vi "Panel Data_File_Init DPT.vi"(0 "Data File Directory":path=path "c:/data", 1 "Test_Title Per TR:":string="HeatUP", 2 "Test Station:":string="1A", 3 "Scale Com Port":refnum<visa-resource-name>="COM1", 5 "Test_Type:":string="HeatUP", 7 "Version In:":string="DGnn", 9 "Supply Voltage:":string(combo), 10 "Flow Computer Info Baro,BTUF,u,Z":string[][](array[string]), 11 "error in (no error)":errorcluster, 12 "File Extension:":string="tmp", 13 "Ambient Temp SetPoint:":string="70") -> (4 "FileName":path, 6 "Header Data Array":string[][](array[string]), 8 "Nominal Load  Weight":string(combo), 14 "Weights Out":T1={"Measured IMC"=7.0, "Actual RMC"=7.0, "RMC (Desired)"=100.0, "Bone Dry Wt(lbs)"=7.0, "Tolerance(%)"=5.0} {"Tolerance(%)" format="%0#_6g"; "Bone Dry Wt(lbs)" format="%03_6g"; "RMC (Desired)" format="%0#_6g"; "Actual RMC" format="%03_6g"; "Measured IMC" format="%0#_6g"}, 15 "error out":errorcluster)   [LabVIEW 2012]
uses:
  Global Test Variables DPT.vi
  <vilib>/Utility/file.llb/Write To Spreadsheet File (string).vi
panel:
  in  "Tab Control 2":enum32{"Test Information"}(tab)
  in  "Model:":string="DGnn"
  in  "Engineer:":string="CraigT."
  in  "Technician:":string
  in  "Comments:":string
  in  "Lab ID:":string="DGnn"
  in  "TR Number:":string="T000000"
  in  "Load Run Number:":string="001"
  in  "Exhaust:":string(combo)="NR"
  in  "Drying Cycle:":string(combo)
  in  "OK":bool
  in  "Serial Number:":string="DGnn"
  in  "Ambient RH:":string="50"
  in  "Build:":string(combo)
  in  "Heat Setting:":string
  in  "Dryness Setting:":string
  in  "Frequency:":string="60 HZ"
  in  "Washer Water \nTemperature ( 60 ± 5°F ):":string="60"
  in  "Tab Control":enum32{"Location Data", "Output Data"}(tab)
  out "Unhandled Error":errorcluster
  out "Filename":string
  in  "Load Definition File":path=path "c:/Work/Loads.ini"
  out "Version:":string="DGnn"
  out "Computer:":string="1A"
  out "Load Type":string(combo)
  out "Empty Dryer Cold Weight":string="HeatUP"
  out "Date:":string="DGnn"
  out "Dryer Type:":string(combo)
  # "Filename Generated"
  # "Trrrrrrrr_uuuuuuuu_WWlb_LLLLLL_aham_xxIMC_tsid_dlr_run nnn_yyyymmdd_hhmm_DPT\nWhere:\nTrrrrrrrr - 8 digit TR #, left padded with 0's\nuuuuuuuu - is LabID number\nWW - Nom Weight\nLLLLLL - Load Type\naham - Restriction\nxx - Nom IMC\ntsid - Test Station\ndlr - Technician\nnnn - Test #\n70 - Nom Ambient Temp\n50 - Nom Ambient RH\nyyyymmddhhmm - day, month as 3 chars, 4 digit year(automatic)\nhhmm - hour and minute (24 hr) test started (automatic)\nDPT - Test Type"
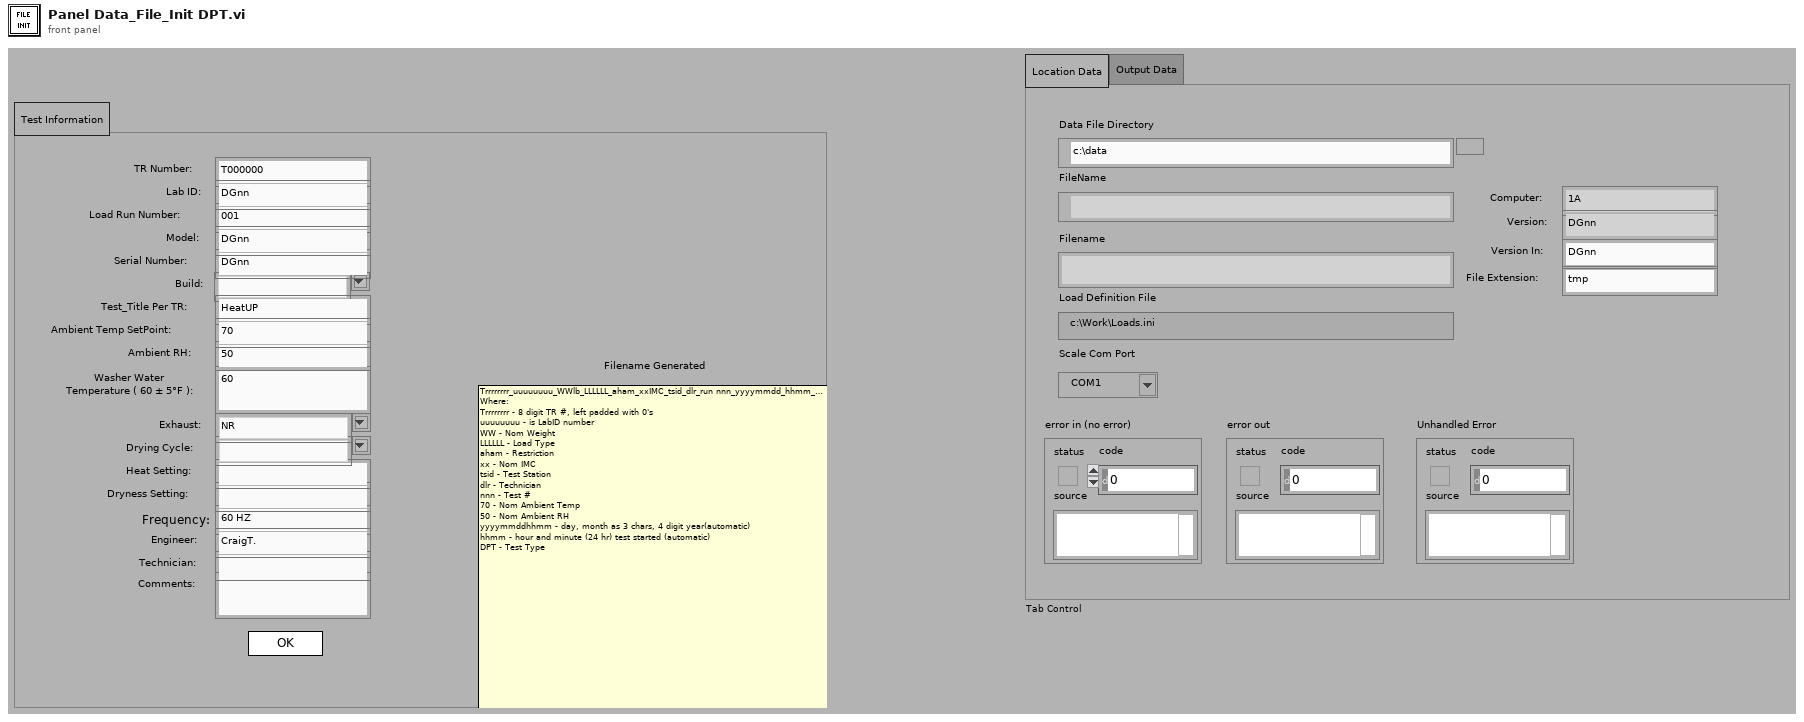
[diagram p1: front panel]
types:
  T1 = cluster{"Measured IMC":dbl, "Actual RMC":dbl, "RMC (Desired)":dbl, "Bone Dry Wt(lbs)":dbl, "Tolerance(%)":dbl}
  T2 = enum32{"invalid app kind", "Development System", "Run Time System", "Student Edition", "Embedded LabVIEW", "Evaluation", "Custom"}
  T3 = enum32{"Invalid", "Standard", "Closed", "Hidden", "Minimized", "Maximized"}
  T4 = cluster{"Core":cluster{"Current VI Reference":refnum<vi>, "Close Panel on Exit?":bool}, "Error Flag":bool, "Weights":cluster{"Measured IMC":dbl, "Actual RMC":dbl, "RMC (Desired)":dbl, "Bone Dry Wt(lbs)":dbl, "Tolerance(%)":dbl}, "Local?":bool}
  T5 = cluster{"Current VI Reference":refnum<vi>, "Close Panel on Exit?":bool}
  T6 = typedef "DPT Global Type.ctl" = cluster{"Test Setup":cluster{"RH Resistor":dbl, "Temp Cal":dbl, "Temp Coeff":dbl, "Power On Threshold":dbl, "MA Filter Size":i32, "Weight Offset":dbl, "Temp Resistor":dbl, "Gas Enabled":bool, "Gas P. Resistor":dbl, "Scale Com":dbl, "W. Samps":i32, "Temp4mA Val":dbl, "Temp20mA Val":dbl, "RH4mA Val":dbl, "RH20mA Val":dbl, "GPres4mA Val":dbl, "Gpres20mA Val":dbl, "Smoothing":bool, "CDAQ":bool, "34970":bool, "34980":bool, "RH-IP":string, "RH-IP2":string, "RH-IP3":string, "CompVolume":dbl, "T45_Coeff.":dbl}, "Agilent Setup":cluster{"Scale Channel":string, "TC Channels":string, "VDC Discrete Channels":string, "RH Chan":string, "Temp Chan":string, "Tscale Channel":string, "RDB Channel":string, "Gas Temperature":string, "Gas Pressure":string, "Barometric Pressure":string, "Gas Feedback Chan":string}, "Directories":cluster{"Work File Directory":path, "Save File Directory":path, "Library Directory":path, "Data Backup Directory":path, "Data Backup Dir Fail":path, "Lab Directory":path}, "Test Information":cluster{"Model:":string, "Temperature:":string, "Engineer:":string, "Technician:":string, "Comments:":string, "Lab ID:":string, "TR Number:":string, "Test Number:":string, "Test Station:":string, "Empty Dryer Cold Weight:":dbl, "Serial Number:":string, "Build:":string, "Dryer Type":string, "Humidity":string, "Test Title per TR:":string}, "cDAQ Array Locations":cluster{"Scale Channel":string, "TC Channels":string, "VDC Discrete Channel":string, "RH Chan":string, "Temp Chan":string, "Tscale Channel":string, "RDB Channel":string, "Gas Temperature":string, "Gas Pressure":string, "Barometric Pressure":string, "Gas Feedback Chan":string}}
  T7 = cluster{"Model:":string, "Temperature:":string, "Engineer:":string, "Technician:":string, "Comments:":string, "Lab ID:":string, "TR Number:":string, "Test Number:":string, "Test Station:":string, "Empty Dryer Cold Weight:":dbl, "Serial Number:":string, "Build:":string, "Dryer Type":string, "Humidity":string, "Test Title per TR:":string}
  T8 = typedef "DOE Audit Data.ctl" = cluster{"Technician":string, "Date":string, "Model":string, "Serial":string, "Total Dry Time(m)":dbl, "Bone Dry Wt":dbl, "Initial Wt":dbl, "Final Wt":dbl, "Initial Ret":dbl, "Final Ret":dbl, "Elect Energy Used":dbl, "Gas Meter Temp":dbl, "Gas Meter Pres":dbl, "Gas Volume":dbl, "Barometer Temp":dbl, "Barometer Pres":dbl, "Gas Corr Fact":dbl, "Cor Gas Vol":dbl, "Gas Heat Val":dbl, "Gas Energy BTU":dbl, "Gas Energy kwh 4%":dbl, "Elect Energy kwh 4%":dbl, "Total  Energy 4%":dbl, "Gas Vol Init":dbl, "Gas Vol Fin":dbl, "Start Time(s)":dbl, "End Time(s)":dbl, "Elect Energy Start":dbl, "Elect Energy End":dbl, "Per Cycle Efficency":dbl, "Annual Consumption":dbl, "Load Cycles":string, "Ambinet Temp":string, "Ambinet RH":string, "Per Cycle Off Mode/Standby Power":dbl, "Total Energy (Gas + Elect)":dbl, "Combined Energy Factor":dbl, "Off Mode Power":dbl, "Exhaust":string, "Washer Water Temperature ( 60 ± 5°F )":string, "Supply Voltage":string, "Reference Temperature (F)":string, "Reference Pressure (psi)":string, "Standby Power":dbl}
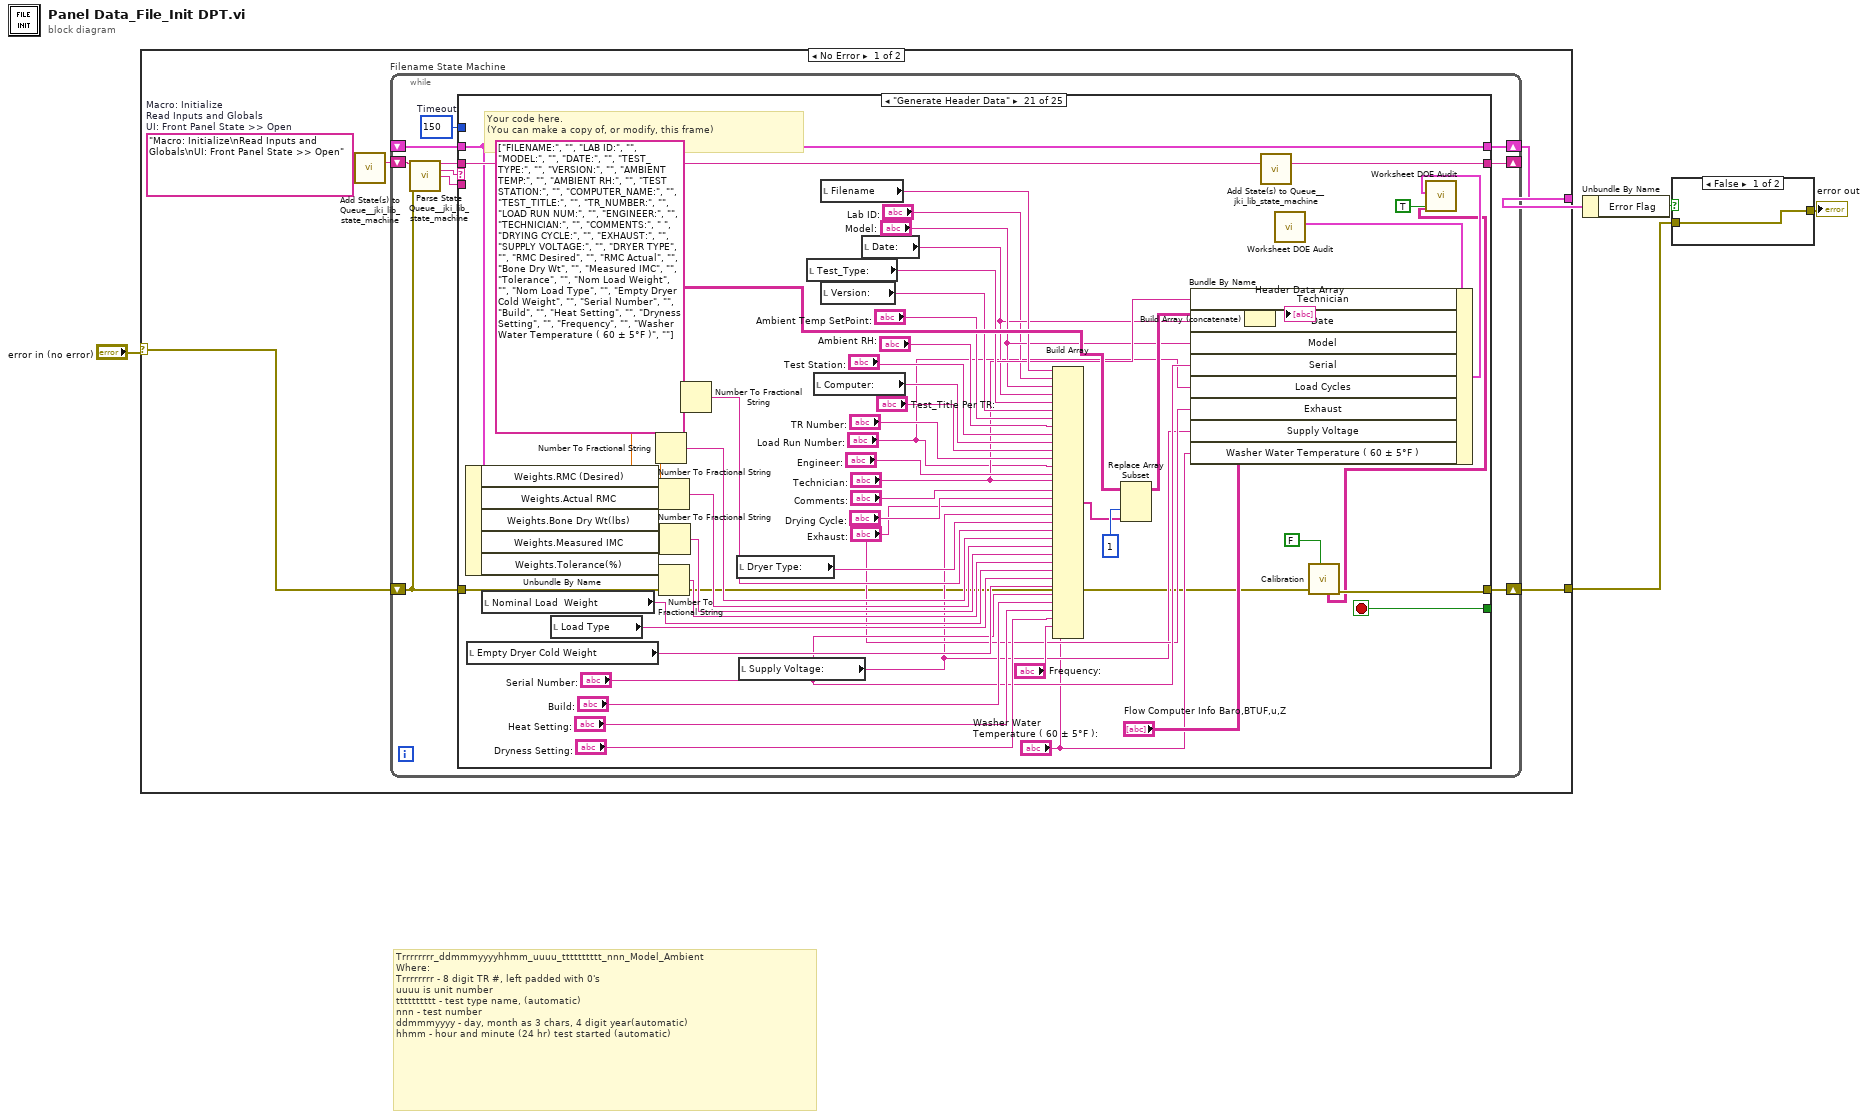
[diagram p0: block diagram]
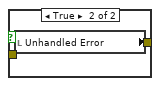
[diagram p2: hidden frame]
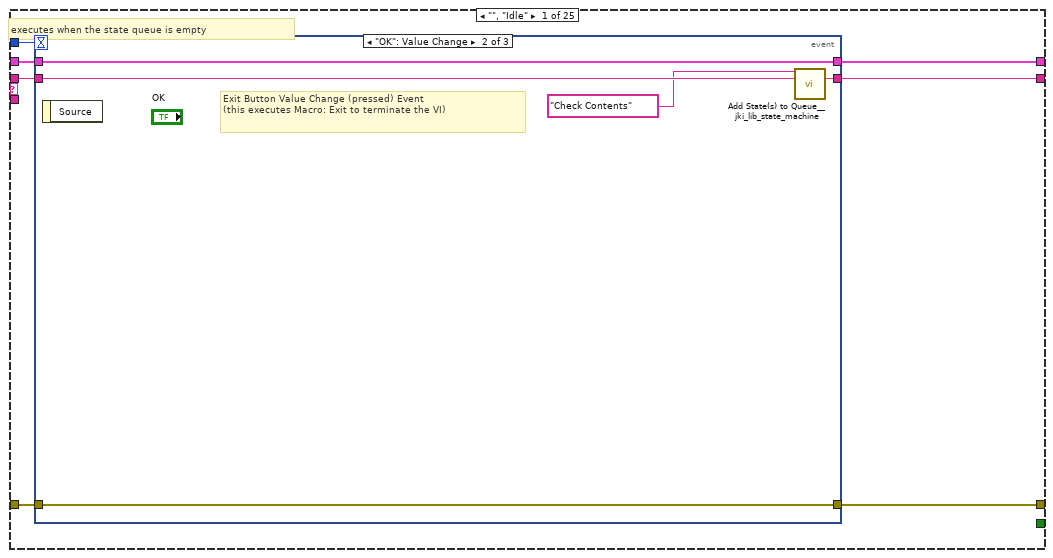
[diagram p3: hidden frame]
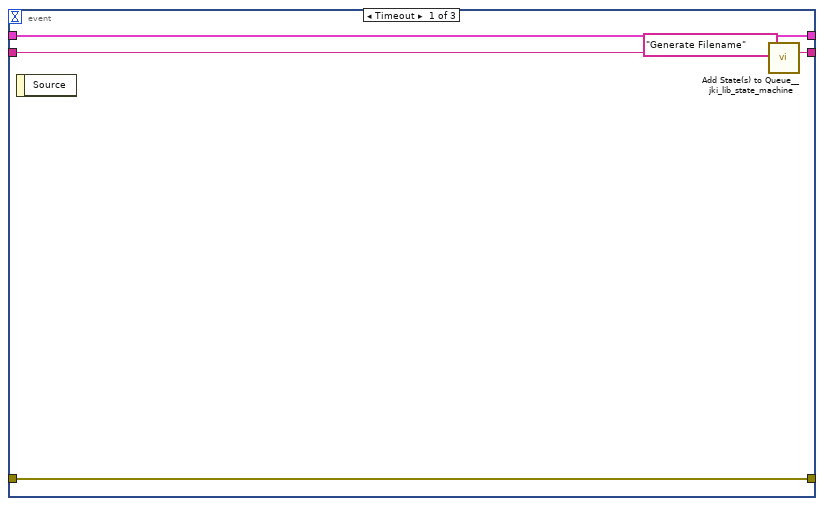
[diagram p4: hidden frame]
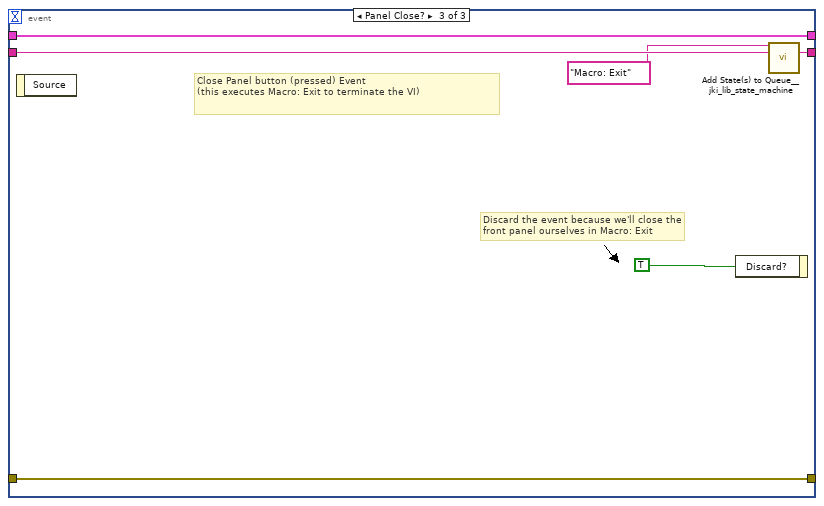
[diagram p5: hidden frame]
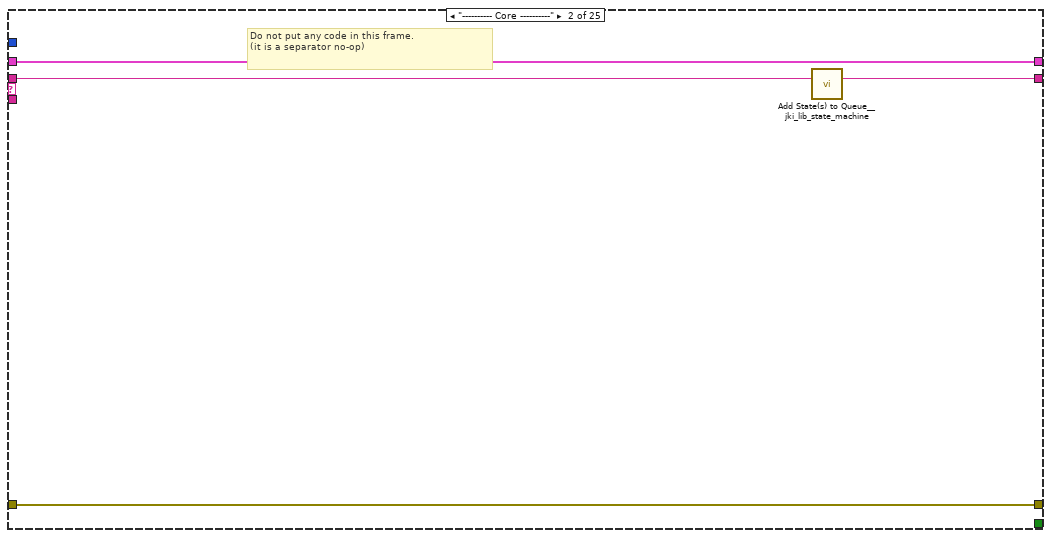
[diagram p6: hidden frame]
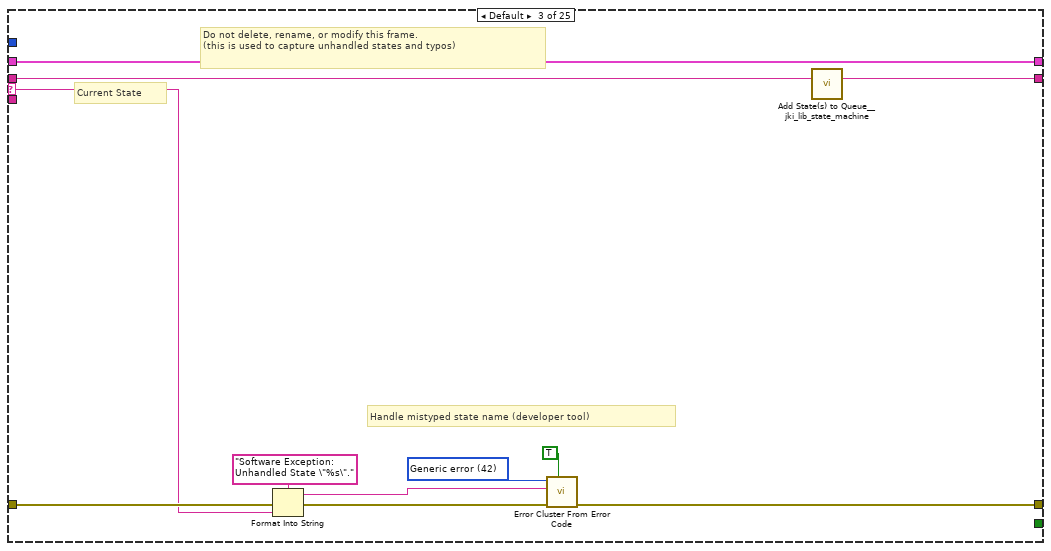
[diagram p7: hidden frame]
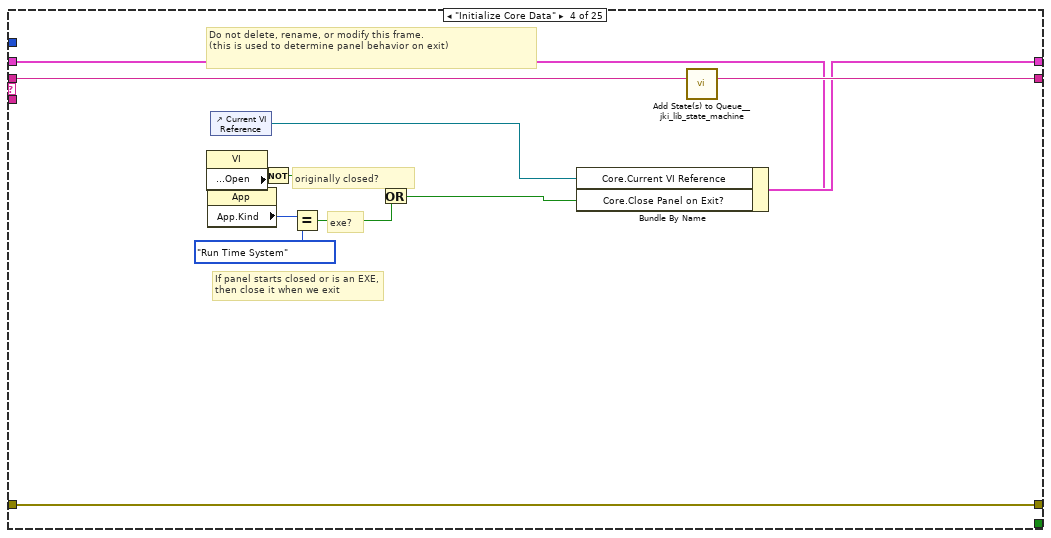
[diagram p8: hidden frame]
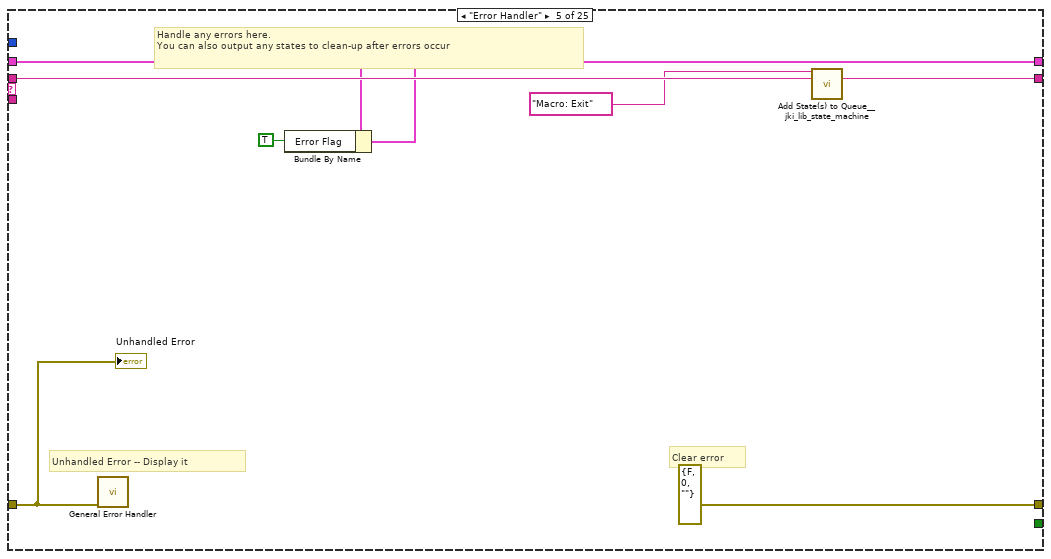
[diagram p9: hidden frame]
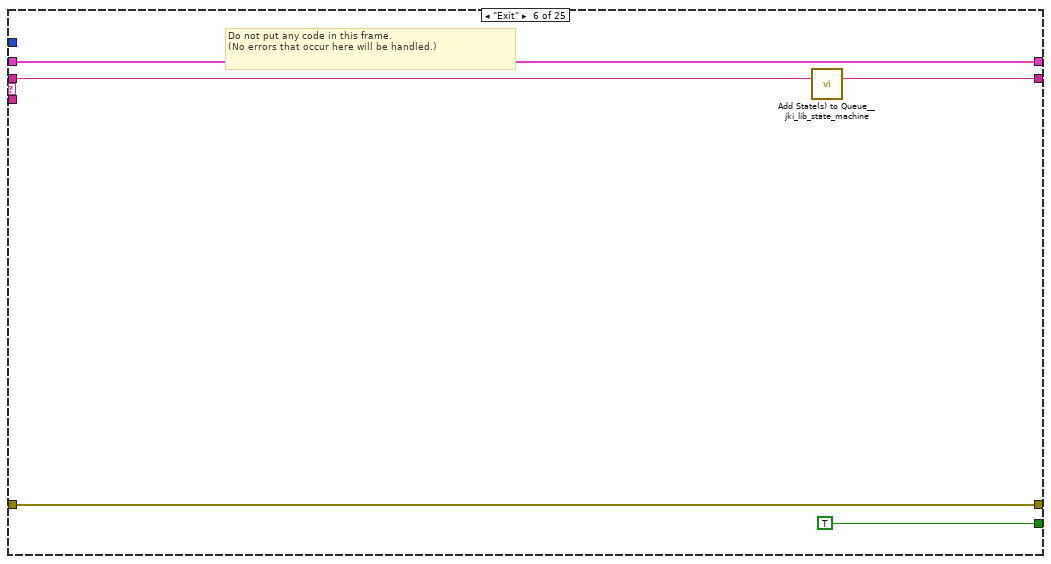
[diagram p10: hidden frame]
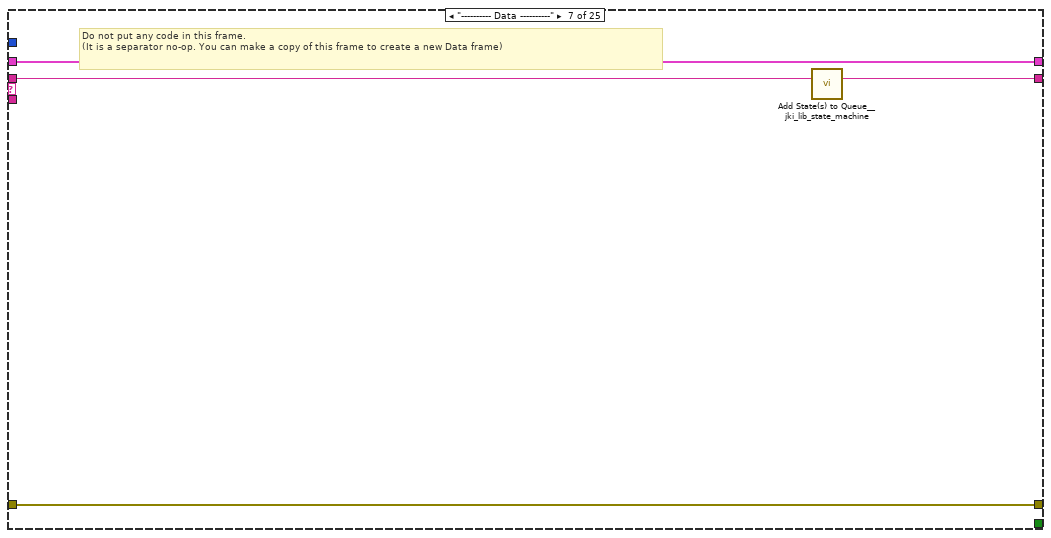
[diagram p11: hidden frame]
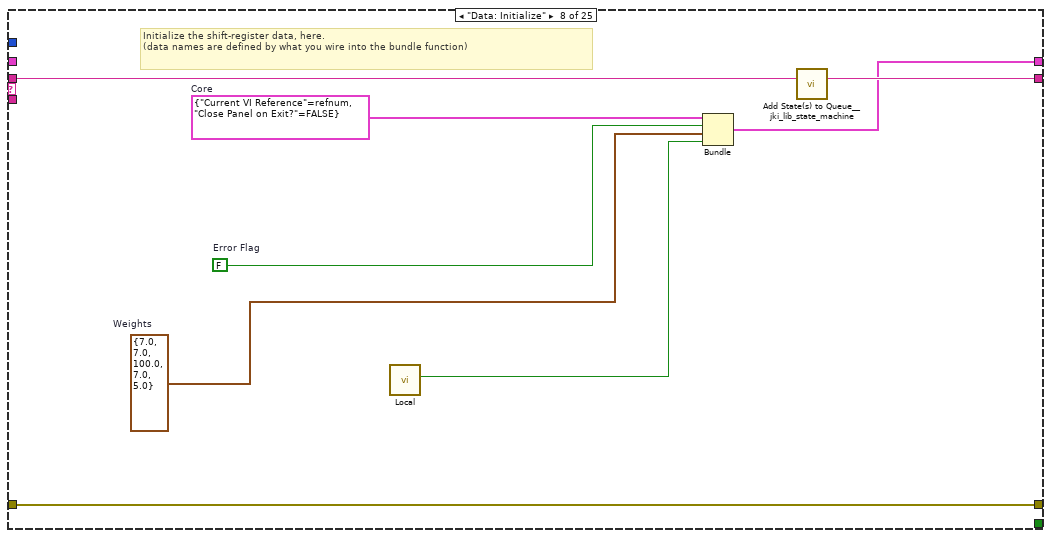
[diagram p12: hidden frame]
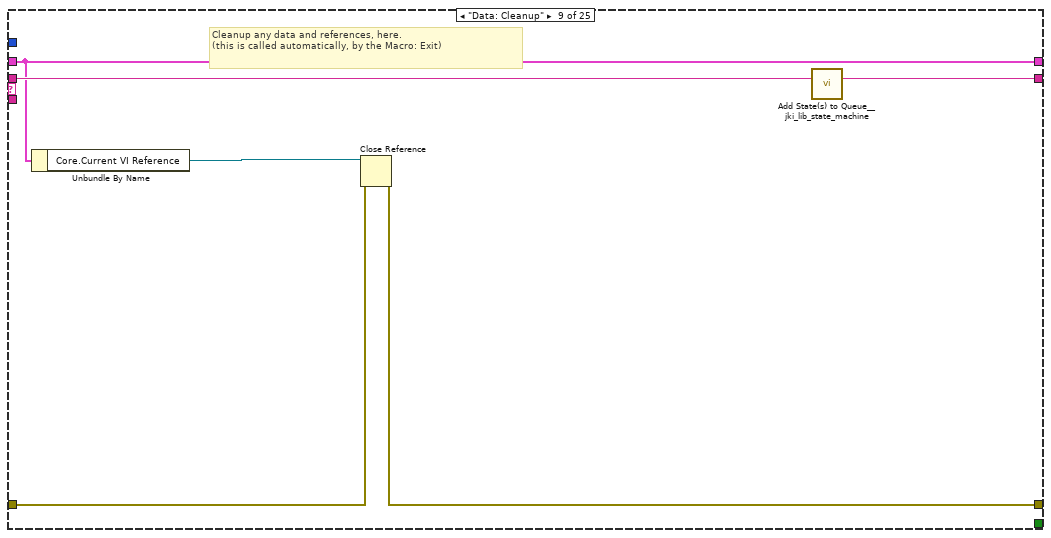
[diagram p13: hidden frame]
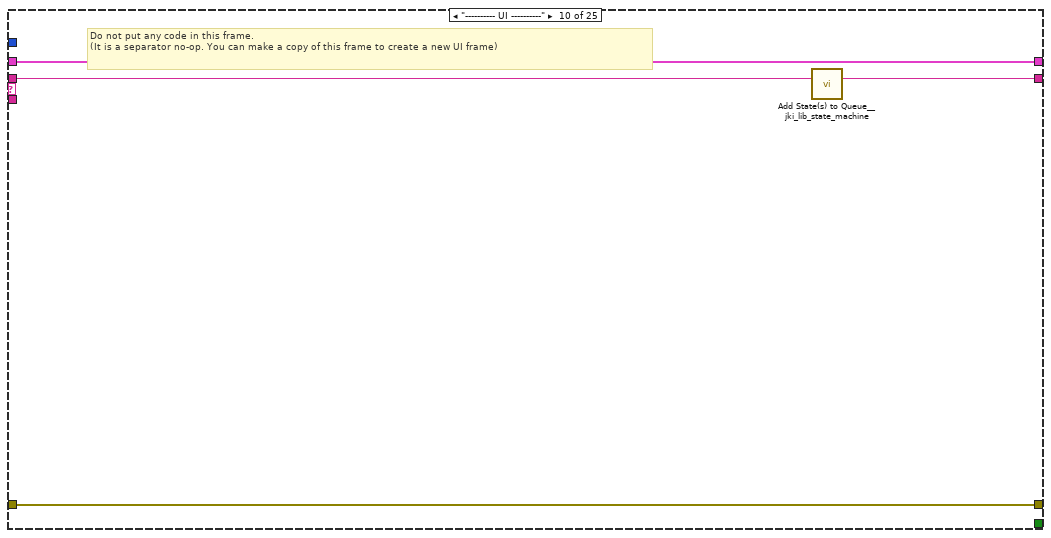
[diagram p14: hidden frame]
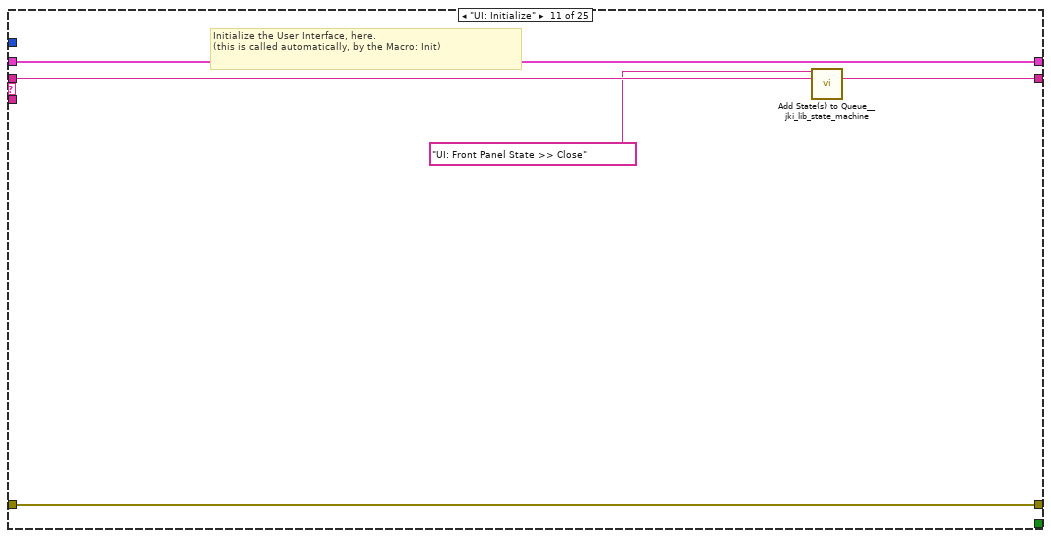
[diagram p15: hidden frame]
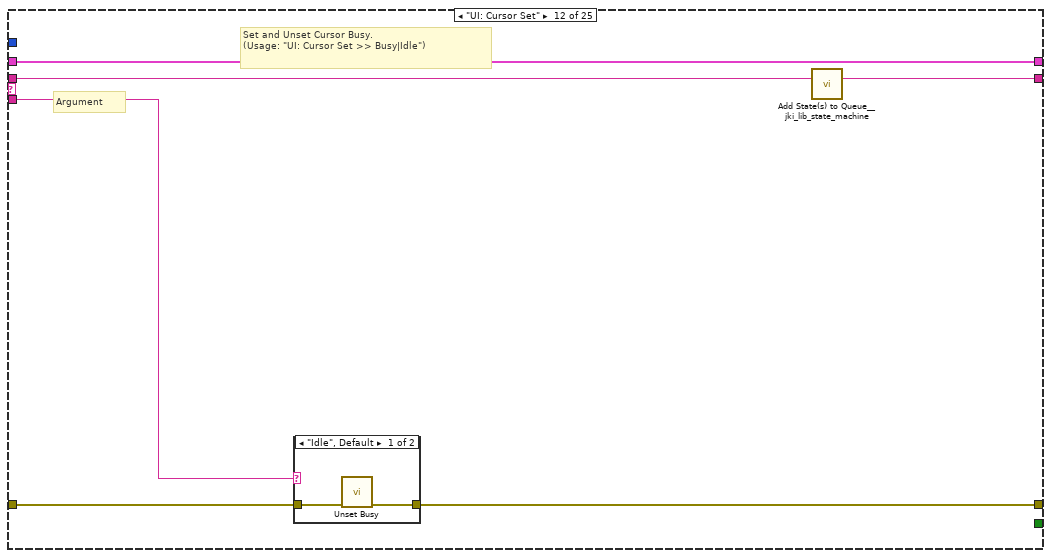
[diagram p16: hidden frame]
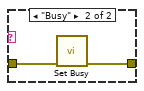
[diagram p17: hidden frame]
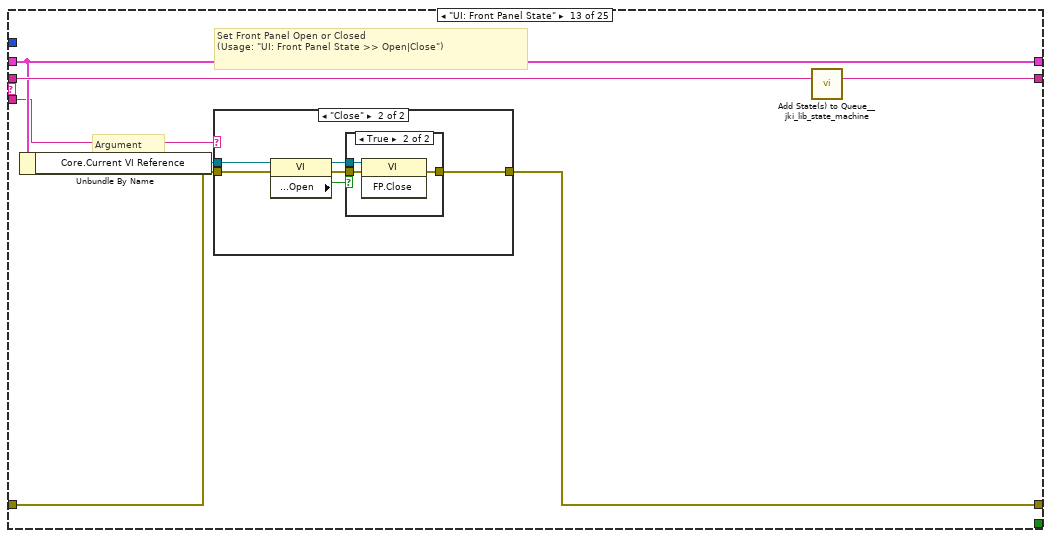
[diagram p18: hidden frame]
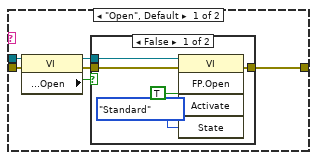
[diagram p19: hidden frame]
diagram:
  # "Trrrrrrrr_ddmmmyyyyhhmm_uuuu_tttttttttt_nnn_Model_Ambient\nWhere:\nTrrrrrrrr - 8 digit TR #, left padded with 0's\nuuuu is unit number\ntttttttttt - test type name, (automatic)\nnnn - test number\nddmmmyyyy - day, month as 3 chars, 4 digit year(automatic)\nhhmm - hour and minute (24 hr) test started (automatic)"
  n1 = case shown="No Error" "error in (no error)" {
    selector: "error in (no error)" -> [w7 w377]
    tunnel: [w8 _] -> w4
    tunnel: [w6 w377] -> w1
    frame No Error {
      w9 = "Macro: Initialize\nRead Inputs and Globals\nUI: Front Panel State >> Open"  # Macro: Initialize Read Inputs and Globals UI: Front Panel State >> Open
      n2 = call <vilib>:"Add State(s) to Queue__jki_lib_state_machine.vi"("State(s) in (\"\")"=w9) -> ("States Out"=w10:string)  [unwired: 14 in]
      n3 = while "Filename State Machine" {
        shift-right: [w14] -> w8
        shift-left: _ -> [w13]
        shift-right: [w17] -> w6
        shift-left: w7 -> [w11]
        shift-right: [w16] -> _
        shift-left: w10 -> [w18]
        stop <- w15 stop-if-true
        w12 = 150  # Timeout
        n4 = call <vilib>:"Parse State Queue__jki_lib_state_machine.vi"("State Queue"=w18, "Error In (no error)"=w11) -> ("Remaining States"=w20:string, "Current State"=w21:string, "Arguments"=w19:string)  [unwired: 11 in]
        n5 = case shown="\"Generate Header Data\"" w21 {
          selector: w21 -> [_ _ w49 _ _ _ _ _ _ _ _ _ _ _ _ _ _ _ _ _ _ _ _ _ _]
          tunnel: w20 -> [w28 w48 w53 w71 w79 w84 w88 w96 w102 w106 w111 w117 w128 w154 w163 w175 w179 w205 w225 w256 w315 w326 w353 w369 w376]
          tunnel: w19 -> [_ _ _ _ _ _ _ _ _ _ _ w112 w122 _ _ _ _ _ _ _ _ _ _ _ _]
          tunnel: w13 -> [w26 w45 w51 w62 w74 w82 w85 _ w97 w103 w109 w115 w124 w151 w160 w172 w176 w202 w222 w254 w300 w323 w340 w366 w371]
          tunnel: [w25 w46 w55 w68 errorcluster {"status"=FALSE, "code"=0, "source"=""} ("error out") w81 w86 w93 w98 w104 w108 w113 w125 w152 w161 w173 w177 w203 w223 w232 w263 w324 w351 w367 w374] -> w17
          tunnel: w11 -> [w24 w46 w54 w68 w76 w81 w86 w93 w99 w104 w108 w114 w126 w152 w161 w173 w177 w203 w223 w233 w264 w324 w351 w367 w374]
          tunnel: [w27 w47 w52 w70 w78 w83 w87 w95 w101 w105 w110 w116 w127 w153 w162 w174 w178 w204 w224 w255 w314 w325 w352 w368 w375] -> w16
          tunnel: [_ _ _ _ _ TRUE _ _ _ _ _ _ _ _ _ _ _ _ _ _ _ _ _ _ _] -> w15
          tunnel: [w23 w45 w51 w69 w73 w82 w85 w94 w97 w103 w109 w115 w124 w151 w160 w172 w176 w202 w222 w254 w300 w323 w340 w365 w371] -> w14
          tunnel: w12 -> [w22 _ _ _ _ _ _ _ _ _ _ _ _ _ _ _ _ _ _ _ _ _ _ _ _]
          frame "", "Idle" {
            # "executes when the state queue is empty"
            n6 = event shown="[1] \"OK\": Value Change" {
              selector: _ -> [_ _ _]
              dyn-events: _ -> [_ _ _]
              timeout: w22 -> [_ _ _]
              tunnel: w28 -> [w33 w38 w44]
              tunnel: [w32 w37 w43] -> w27
              tunnel: w26 -> [w30 w35 w41]
              tunnel: [w31 w36 w42] -> w25
              tunnel: w24 -> [w31 w36 w42]
              tunnel: [w30 w35 w41] -> w23
              event Timeout {
                n7 = event-data() -> ()  [unwired: 1 in, 1 out]
                n8 = call <vilib>:"Add State(s) to Queue__jki_lib_state_machine.vi"("State(s) in Front (\"\")"="Generate Filename" ("State(s) in Front (\"\")"), "State(s) in (\"\")"=w33) -> ("States Out"=w32:string)  [unwired: 13 in]
              }
              event "OK": Value Change {
                # "Exit Button Value Change (pressed) Event\n(this executes Macro: Exit to terminate the VI)"
                n9 = event-data() -> ()  [unwired: 1 in, 1 out]
                n10 = call <vilib>:"Add State(s) to Queue__jki_lib_state_machine.vi"("State(s) in Front (\"\")"="Check Contents", "State(s) in (\"\")"=w38) -> ("States Out"=w37:string)  [unwired: 13 in]
              }
              event Panel Close? {
                # "Discard the event because we'll close the front panel ourselves in Macro: Exit"
                # "Close Panel button (pressed) Event\n(this executes Macro: Exit to terminate the VI)"
                n11 = event-data() -> ()  [unwired: 1 in, 1 out]
                n12 = event-data("Discard?"=TRUE) -> ()  [unwired: 1 in, 1 out]
                n13 = call <vilib>:"Add State(s) to Queue__jki_lib_state_machine.vi"("State(s) in Front (\"\")"="Macro: Exit", "State(s) in (\"\")"=w44) -> ("States Out"=w43:string)  [unwired: 13 in]
              }
            }
          }
          frame "---------- Core ----------" {
            # "Do not put any code in this frame.\n(it is a separator no-op)"
            n14 = call <vilib>:"Add State(s) to Queue__jki_lib_state_machine.vi"("State(s) in (\"\")"=w48) -> ("States Out"=w47:string)  [unwired: 14 in]
          }
          frame Default {
            w58 = 42 items=["No error", "Argument error", "Memory is full", "Out of zone", "End of file", "File already open", "Generic file I/O error", "File not found", "File permission error", "Disk is full", "Duplicate path", "Too many files open", "System feature not enabled", "Resource file not found", "Cannot add resource", "Resource not found", "Image not found", "Image memory error", "Pen does not exist", "Config type invalid", "Config token not found", "Config parse error", "Config memory error", "Bad external code format", "Bad external code offset", "External code not present", "Null window", "Destroy window error", "Null menu", "Print aborted", "Bad print record", "Print driver error", "Windows error during printing", "Memory error during printing", "Print dialog error", "Generic print error", "Invalid device refnum", "Device not found", "Device parameter error", "Device unit error", "Cannot open device", "Device call aborted", "Generic error", "Cancelled by user", "Object ID too low", "Object ID too high", "Object not in heap", "Unknown heap", "Unknown object (invalid DefProc)", "Unknown object (DefProc not in table)", "Message out of range", "Invalid (null) method", "Unknown message", "Manager call not supported", "Bad address", "Network operation in progress", "Network operation timed out", "Connection is busy", "Network attribute not supported", "Network error", "Address in use", "System out of memory", "Connection aborted", "Connection refused", "Not connected", "Already connected", "Connection closed", "Initialization error (interapplication manager)", "Bad occurrence", "Wait on unbound occurrence handler", "Occurrence queue overflow", "Datalog type conflict", "Unused", "Unrecognized type (interapplication manager)", "Memory corrupt", "Failed to make temporary DLL", "Old CIN version", "Drag socket not found", "Failed to load drop-object", "Failed to register OLE object", "Failed to release OLE object", "Format specifier type mismatch", "Unknown format specifier", "Too few format specifiers", "Too many format specifiers", "Scan failed", "Newer CIN version", "Error converting to variant", "Runtime menu error", "Password tampered", "Variant attribute not found", "Incompatible variant data type", "Event data is not available", "Event Store is not present", "Occurrence is not found", "Event Queue is not created", "Event info is not available", "Refnum passed is NULL", "Error retrieving Class GUID", "Error retrieving CoClass GUID", "Error retrieving TypeLib GUID.", "Bad built application magic bytes.", "Specific driver is different from the specific driver associated with the Logical Name.", "There is no session opened to the class driver.", "Max Error", "MAX - Error with config objects", "MAX - Error loading configuration", "MAX - Group not supported"]
            # "Current State"
            # "Do not delete, rename, or modify this frame.\n(this is used to capture unhandled states and typos)"
            # "Handle mistyped state name (developer tool)"
            n15 = Format Into String(format string="Software Exception: Unhandled State \"%s\"." ("message"), error in=w54, w49) -> (resulting string=w57:string, error out=w56:errorcluster)  [unwired: 1 in]
            n16 = call <vilib>:"Error Cluster From Error Code.vi"("show call chain? (False)"=TRUE, "error in (no error)"=w56, "error message (\"\")"=w57, "error code (0)"=w58) -> ("error out"=w55:errorcluster)  [unwired: 5 in]
            n17 = call <vilib>:"Add State(s) to Queue__jki_lib_state_machine.vi"("State(s) in (\"\")"=w53) -> ("States Out"=w52:string)  [unwired: 14 in]
          }
          frame "Initialize Core Data" {
            # "Do not delete, rename, or modify this frame.\n(this is used to determine panel behavior on exit)"
            # "originally closed?"
            # "exe?"
            # "If panel starts closed or is an EXE, then close it when we exit"
            n18 = property class="VI"() -> ("Front Panel.Open"=w67:bool)  [unwired: 2 in, 2 out]
            n19 = property class="App"() -> ("App.Kind"=w66:T2)  [unwired: 2 in, 2 out]
            n20 = control-ref of="Current VI Reference"() -> (w60:refnum<vi>)
            n21 = Not(x=w67) -> (.not. x?=w64:bool)
            n22 = Equal?(x=w66, y=T2."Run Time System" ("Application:Kind")) -> (x = y?=w63:bool)
            n23 = Or(x=w64, y=w63) -> (x .or. y?=w61:bool)
            n24 = Bundle By Name(cluster=w62, "Core.Current VI Reference"=w60, "Core.Close Panel on Exit?"=w61) -> (w69:T4)
            n25 = call <vilib>:"Add State(s) to Queue__jki_lib_state_machine.vi"("State(s) in (\"\")"=w71) -> ("States Out"=w70:string)  [unwired: 14 in]
          }
          frame "Error Handler" {
            # "Unhandled Error -- Display it"
            # "Handle any errors here.\nYou can also output any states to clean-up after errors occur"
            # "Clear error"
            n26 = call <vilib>:"General Error Handler.vi"("error in (no error)"=w76) -> ()  [unwired: 10 in, 5 out]
            n27 = Bundle By Name(cluster=w74, "Error Flag"=TRUE) -> (w73:T4)
            n28 = call <vilib>:"Add State(s) to Queue__jki_lib_state_machine.vi"("State(s) in Front (\"\")"="Macro: Exit", "State(s) in (\"\")"=w79) -> ("States Out"=w78:string)  [unwired: 13 in]
            "Unhandled Error" <- w76
          }
          frame "Exit" {
            # "Do not put any code in this frame.\n(No errors that occur here will be handled.)"
            n29 = call <vilib>:"Add State(s) to Queue__jki_lib_state_machine.vi"("State(s) in (\"\")"=w84) -> ("States Out"=w83:string)  [unwired: 14 in]
          }
          frame "---------- Data ----------" {
            # "Do not put any code in this frame.\n(It is a separator no-op. You can make a copy of this frame to create a new Data frame)"
            n30 = call <vilib>:"Add State(s) to Queue__jki_lib_state_machine.vi"("State(s) in (\"\")"=w88) -> ("States Out"=w87:string)  [unwired: 14 in]
          }
          frame "Data: Initialize" {
            w90 = T1 {"Measured IMC"=7.0, "Actual RMC"=7.0, "RMC (Desired)"=100.0, "Bone Dry Wt(lbs)"=7.0, "Tolerance(%)"=5.0}  # Weights
            w91 = T5 {"Current VI Reference"=refnum, "Close Panel on Exit?"=FALSE}  # Core
            w92 = FALSE  # Error Flag
            # "Initialize the shift-register data, here.\n(data names are defined by what you wire into the bundle function)"
            n31 = call "Local.vi"() -> ("Local?"=w89:bool)  [unwired: 11 in]
            n32 = Bundle("Core"=w91, "Error Flag"=w92, "Weights"=w90, "Local?"=w89) -> (w94:T4)  [unwired: 1 in]
            n33 = call <vilib>:"Add State(s) to Queue__jki_lib_state_machine.vi"("State(s) in (\"\")"=w96) -> ("States Out"=w95:string)  [unwired: 14 in]
          }
          frame "Data: Cleanup" {
            # "Cleanup any data and references, here.\n(this is called automatically, by the Macro: Exit)"
            n34 = Unbundle By Name(w97) -> ("Core.Current VI Reference"=w100:refnum<vi>)
            n35 = Close Reference(reference=w100, error in (no error)=w99) -> (error out=w98:errorcluster)
            n36 = call <vilib>:"Add State(s) to Queue__jki_lib_state_machine.vi"("State(s) in (\"\")"=w102) -> ("States Out"=w101:string)  [unwired: 14 in]
          }
          frame "---------- UI ----------" {
            # "Do not put any code in this frame.\n(It is a separator no-op. You can make a copy of this frame to create a new UI frame)"
            n37 = call <vilib>:"Add State(s) to Queue__jki_lib_state_machine.vi"("State(s) in (\"\")"=w106) -> ("States Out"=w105:string)  [unwired: 14 in]
          }
          frame "UI: Initialize" {
            # "Initialize the User Interface, here.\n(this is called automatically, by the Macro: Init)"
            n38 = call <vilib>:"Add State(s) to Queue__jki_lib_state_machine.vi"("State(s) in Front (\"\")"="UI: Front Panel State >> Close", "State(s) in (\"\")"=w111) -> ("States Out"=w110:string)  [unwired: 13 in]
          }
          frame "UI: Cursor Set" {
            # "Argument"
            # "Set and Unset Cursor Busy.\n(Usage: \"UI: Cursor Set >> Busy|Idle\")"
            n39 = case shown="\"Idle\", Default" w112 {
              tunnel: w114 -> [w119 w121]
              tunnel: [w118 w120] -> w113
              frame "Idle", Default {
                n40 = call <vilib>:"Unset Busy.vi"("error in (no error)"=w119) -> ("error out"=w118:errorcluster)  [unwired: 10 in]
              }
              frame "Busy" {
                n41 = call <vilib>:"Set Busy.vi"("error in (no error)"=w121) -> ("error out"=w120:errorcluster)  [unwired: 9 in, 1 out]
              }
            }
            n42 = call <vilib>:"Add State(s) to Queue__jki_lib_state_machine.vi"("State(s) in (\"\")"=w117) -> ("States Out"=w116:string)  [unwired: 14 in]
          }
          frame "UI: Front Panel State" {
            # "Argument"
            # "Set Front Panel Open or Closed\n(Usage: \"UI: Front Panel State >> Open|Close\")"
            n43 = Unbundle By Name(w124) -> ("Core.Current VI Reference"=w123:refnum<vi>)
            n44 = case shown="\"Close\"" w122 {
              tunnel: w126 -> [w132 w145]
              tunnel: [w134 w146] -> w125
              tunnel: w123 -> [w133 w143]
              frame "Open", Default {
                n45 = property class="VI"(reference=w133, error in=w132) -> (reference out=w130:refnum<vi>, error out=w131:errorcluster, "Front Panel.Open"=w129:bool)
                n46 = case shown="False" w129 {
                  tunnel: [w137 w140] -> w134
                  tunnel: w131 -> [w136 w140]
                  tunnel: w130 -> [w135 _]
                  frame False {
                    n47 = invoke class="VI" method="FP.Open"(reference=w135, error in=w136, "Activate"=TRUE, "State"=T3."Standard") -> (error out=w137:errorcluster)  [unwired: 1 in, 4 out]
                  }
                  frame True {
                  }
                }
              }
              frame "Close" {
                n48 = property class="VI"(reference=w143, error in=w145) -> (reference out=w142:refnum<vi>, error out=w144:errorcluster, "Front Panel.Open"=w141:bool)
                n49 = case shown="True" w141 {
                  tunnel: [w147 w150] -> w146
                  tunnel: w144 -> [w147 w149]
                  tunnel: w142 -> [_ w148]
                  frame False {
                  }
                  frame True {
                    n50 = invoke class="VI" method="FP.Close"(reference=w148, error in=w149) -> (error out=w150:errorcluster)  [unwired: 1 in, 2 out]
                  }
                }
              }
            }
            n51 = call <vilib>:"Add State(s) to Queue__jki_lib_state_machine.vi"("State(s) in (\"\")"=w128) -> ("States Out"=w127:string)  [unwired: 14 in]
          }
          frame "---------- Macro ----------" {
            # "Do not put any code in this frame.\n(It is a separator no-op. You can make a copy of this frame to create a new Macro frame)"
            n52 = call <vilib>:"Add State(s) to Queue__jki_lib_state_machine.vi"("State(s) in (\"\")"=w154) -> ("States Out"=w153:string)  [unwired: 14 in]
          }
          frame "Macro: Initialize" {
            # "Initialization Macro\n(This is called once, when the VI starts)"
            n53 = property on="OK" class="Bool"("Key Focus"=FALSE) -> ()  [unwired: 2 in, 2 out]
            n54 = local write "Drying Cycle:"("" ("Drying Cycle:")) -> ()
            n55 = local write "Exhaust:"("" ("Exhaust:")) -> ()
            n56 = local write "Dryer Type:"("" ("Dryer Type:")) -> ()
            n57 = call <vilib>:"Add State(s) to Queue__jki_lib_state_machine.vi"("State(s) in Front (\"\")"="Data: Initialize\nInitialize Core Data\nUI: Initialize", "State(s) in (\"\")"=w163) -> ("States Out"=w162:string)  [unwired: 13 in]
          }
          frame "Macro: Exit" {
            # "Exit Macro\n(This is called once, when the VI exits)"
            n58 = Unbundle By Name(w172) -> ("Core.Close Panel on Exit?"=w171:bool, "Local?"=w164:bool)
            n59 = Compound Arithmetic op=AND(w171, invert w164) -> (w165:bool)
            n60 = Select(t="UI: Front Panel State >> Close", s=w165, f="") -> (s? t:f=w168:string)
            n61 = call <vilib>:"Add State(s) to Queue__jki_lib_state_machine.vi"("State(s) in (\"\")"=w168, "State(s) at Back (\"\")"="Data: Cleanup\nExit") -> ("States Out"=w166:string)  [unwired: 13 in]
            n62 = call <vilib>:"Add State(s) to Queue__jki_lib_state_machine.vi"("State(s) in Front (\"\")"=w166, "State(s) in (\"\")"=w175) -> ("States Out"=w174:string)  [unwired: 13 in]
          }
          frame "---------- New Category ----------" {
            # "Template Separator\n(You can make a copy of, or modify, this frame)"
            n63 = call <vilib>:"Add State(s) to Queue__jki_lib_state_machine.vi"("State(s) in (\"\")"=w179) -> ("States Out"=w178:string)  [unwired: 14 in]
          }
          frame "Read Inputs and Globals" {
            n64 = global read "Global Test Variables DPT.vi" "Globals for Dryer Performance Test"() -> (w197:T6)
            n65 = call "IP and Computer Name.vi"() -> ("Computer Name"=→"Computer:":string)  [unwired: 10 in, 1 out]
            n66 = Unbundle By Name(w197) -> ("Test Information"=w196:T7)
            n67 = Unbundle(w196) -> ("Model:"=w195:string, "Temperature:"=w187:string, "Engineer:"=w194:string, "Technician:"=w193:string, "Comments:"=w192:string, "Lab ID:"=w191:string, "TR Number:"=w190:string, "Test Number:"=w189:string, "Test Station:"=w188:string, "Empty Dryer Cold Weight:"=w184:dbl, "Serial Number:"=w186:string, "Build:"=w185:string, "Dryer Type"=→"Dryer Type:":string, "Humidity"=w181:string, "Test Title per TR:"=w180:string)
            n68 = local write "Comments:"(w192) -> ()
            n69 = local write "Technician:"(w193) -> ()
            n70 = local write "Test Station:"(w188) -> ()
            n71 = local write "Load Run Number:"(w189) -> ()
            n72 = local write "Ambient Temp SetPoint:"(w187) -> ()
            n73 = local write "Serial Number:"(w186) -> ()
            n74 = Format Date/Time String(time format string (%c)="%Y%m%d_%H%M") -> (date/time string=→"Date:":string)  [unwired: 2 out]
            n75 = local write "Test_Title Per TR:"(w180) -> ()
            n76 = local write "Lab ID:"(w191) -> ()
            n77 = local write "TR Number:"(w190) -> ()
            n78 = local write "Build:"(w185) -> ()
            n79 = local write "Ambient RH:"(w181) -> ()
            n80 = local write "Engineer:"(w194) -> ()
            n81 = local write "Model:"(w195) -> ()
            n82 = Number To Fractional String(number=w184) -> (F-format string=→"Empty Dryer Cold Weight":string)  [unwired: 3 in]
            n83 = call <vilib>:"Add State(s) to Queue__jki_lib_state_machine.vi"("State(s) in (\"\")"=w205) -> ("States Out"=w204:string)  [unwired: 14 in]
            "Version:" <- "Version In:"
          }
          frame "Write Globals" {
            # "Your code here.\n(You can make a copy of, or modify, this frame)"
            n84 = local read "Comments:"() -> (w214:string)
            n85 = local read "Technician:"() -> (w215:string)
            n86 = global read "Global Test Variables DPT.vi" "Globals for Dryer Performance Test"() -> (w211:T6)
            n87 = local read "Test_Title Per TR:"() -> (w208:string)
            n88 = local read "Serial Number:"() -> (w206:string)
            n89 = local read "TR Number:"() -> (w213:string)
            n90 = local read "Test Station:"() -> (w212:string)
            n91 = local read "Ambient RH:"() -> (w207:string)
            n92 = local read "Engineer:"() -> (w216:string)
            n93 = local read "Ambient Temp SetPoint:"() -> (w217:string)
            n94 = local read "Load Run Number:"() -> (w219:string)
            n95 = local read "Model:"() -> (w218:string)
            n96 = local read "Lab ID:"() -> (w220:string)
            n97 = Unbundle By Name(w211) -> ("Test Information"=w221:T7)
            n98 = Bundle By Name(cluster=w221, "Model:"=w218, "Temperature:"=w217, "Engineer:"=w216, "Technician:"=w215, "Comments:"=w214, "Lab ID:"=w220, "TR Number:"=w213, "Test Number:"=w219, "Test Station:"=w212, "Humidity"=w207, "Test Title per TR:"=w208, "Serial Number:"=w206) -> (w210:T7)
            n99 = Bundle By Name(cluster=w211, "Test Information"=w210) -> (w209:T6)
            n100 = global write "Global Test Variables DPT.vi" "Globals for Dryer Performance Test"(w209) -> ()
            n101 = call <vilib>:"Add State(s) to Queue__jki_lib_state_machine.vi"("State(s) in (\"\")"=w225) -> ("States Out"=w224:string)  [unwired: 14 in]
          }
          frame "Generate Filename" {
            # "Trrrrrrrr_uuuuuuuu_WWlb_LLLLLL_aham_xxIMC_tsid_dlr_run nnn_70,50_yyyymmdd_hhmm_DPT\nWhere:\nTrrrrrrrr - 8 digit TR #, left padded with 0's\nuuuuuuuu - is unit number\nWW - Nom Weight\nLLLLLL - Load Type\naham - Restriction\nxx - Nom IMC\ntsid - Test Station\ndlr - Technician\nnnn - Test #\n70 - Nom Ambient Temp\n50 - Nom Ambient RH\nyyyymmddhhmm - day, month as 3 chars, 4 digit year(automatic)\nhhmm - hour and minute (24 hr) test started (automatic)\nDPT - Test Type"
            # "Your code here.\n(You can make a copy of, or modify, this frame)"
            n102 = local read "Ambient Temp SetPoint:"() -> (w249:string)
            n103 = local read "Nominal Load  Weight"() -> (w238:string)
            n104 = local read "Load Run Number:"() -> (w248:string)
            n105 = local read "Weights Out"() -> (w245:T1)
            n106 = local read "Technician:"() -> (w247:string)
            n107 = local read "Test Station:"() -> (w246:string)
            n108 = local read "Load Type"() -> (w239:string)
            n109 = local read "TR Number:"() -> (w252:string)
            n110 = local read "Lab ID:"() -> (w237:string)
            n111 = local read "Date:"() -> (w250:string)
            n112 = local read "Exhaust:"() -> (w240:string)
            n113 = Unbundle By Name(w245) -> ("RMC (Desired)"=w244:dbl)
            n114 = Number To Fractional String(number=w244, width (-)=i16 2, precision (6)=i16 0) -> (F-format string=w243:string)  [unwired: 1 in]
            n115 = Format Into String(format string="%09s_%08s_%2.2slb_%06.6s_%04.4s_%03.3sIMC_%4.4s_%03.3s_run %3.3s_%s_%13.13s_DPT.%3.3s", w252, w237, w238, w239, w240, w243, w246, w247, w248, w249, w250, "File Extension:") -> (resulting string=w229:string)  [unwired: 2 in, 1 out]
            "Filename" <- w229
            n116 = Path To String(path="Data File Directory") -> (string=w227:string)
            n117 = Build Path(base path="Data File Directory", name or relative path=w229) -> (appended path=w235:path)
            "FileName" <- w235
            n118 = Equal?(x=w235, y=path "") -> (x = y?=w234:bool)
            n119 = Concatenate Strings("Error for Filename: " ("source"), w229, " Directory: " ("source"), w227) -> (w226:string)
            n120 = case shown="True" w234 {
              tunnel: w233 -> [w257 _]
              tunnel: [w257 w259] -> w232
              tunnel: w226 -> [_ w258]
              frame False {
              }
              frame True {
                n121 = Bundle By Name(cluster=errorcluster {"status"=TRUE, "code"=-8074, "source"=""} ("error IO"), "source"=w258) -> (w259:errorcluster)
              }
            }
            n122 = call <vilib>:"Add State(s) to Queue__jki_lib_state_machine.vi"("State(s) in (\"\")"=w256) -> ("States Out"=w255:string)  [unwired: 14 in]
          }
          frame "Generate Header Data" {
            # "Your code here.\n(You can make a copy of, or modify, this frame)"
            n123 = Unbundle By Name(w300) -> ("Weights.RMC (Desired)"=w299:dbl, "Weights.Actual RMC"=w298:dbl, "Weights.Bone Dry Wt(lbs)"=w297:dbl, "Weights.Measured IMC"=w296:dbl, "Weights.Tolerance(%)"=w291:dbl)
            n124 = local read "Empty Dryer Cold Weight"() -> (w287:string)
            n125 = local read "Nominal Load  Weight"() -> (w289:string)
            n126 = local read "Load Type"() -> (w288:string)
            n127 = Number To Fractional String(number=w298) -> (F-format string=w294:string)  [unwired: 3 in]
            n128 = Number To Fractional String(number=w297) -> (F-format string=w293:string)  [unwired: 3 in]
            n129 = Number To Fractional String(number=w291) -> (F-format string=w290:string)  [unwired: 3 in]
            n130 = Number To Fractional String(number=w296) -> (F-format string=w292:string)  [unwired: 3 in]
            n131 = Number To Fractional String(number=w299) -> (F-format string=w295:string)  [unwired: 3 in]
            n132 = local read "Dryer Type:"() -> (w283:string)
            n133 = local read "Supply Voltage:"() -> (w266:string)
            n134 = local read "Test_Type:"() -> (w309:string)
            n135 = local read "Computer:"() -> (w306:string)
            n136 = local read "Filename"() -> (w310:string)
            n137 = local read "Version:"() -> (w308:string)
            n138 = local read "Date:"() -> (w274:string)
            n139 = Build Array(w310, "Lab ID:", "Model:", w274, w309, w308, "Ambient Temp SetPoint:", "Ambient RH:", "Test Station:", w306, "Test_Title Per TR:", "TR Number:", "Load Run Number:", "Engineer:", "Technician:", "Comments:", "Drying Cycle:", "Exhaust:", w266, w283, w295, w294, w293, w292, w290, w289, w288, w287, "Serial Number:", "Build:", "Heat Setting:", "Dryness Setting:", "Frequency:", "Washer Water \nTemperature ( 60 ± 5°F ):") -> (w312:string[])
            n140 = Replace Array Subset(array=string[][] [["FILENAME:", ""], ["LAB ID:", ""], ["MODEL:", ""], ["DATE:", ""], ["TEST_TYPE:", ""], ["VERSION:", ""], ["AMBIENT TEMP:", ""], ["AMBIENT RH:", ""], ["TEST STATION:", ""], ["COMPUTER_NAME:", ""], ["TEST_TITLE:", ""], ["TR_NUMBER:", ""], ["LOAD RUN NUM:", ""], ["ENGINEER:", ""], ["TECHNICIAN:", ""], ["COMMENTS:", " "], ["DRYING CYCLE:", ""], ["EXHAUST:", ""], ["SUPPLY VOLTAGE:", ""], ["DRYER TYPE", ""], ["RMC Desired", ""], ["RMC Actual", ""], ["Bone Dry Wt", ""], ["Measured IMC", ""], ["Tolerance", ""], ["Nom Load Weight", ""], ["Nom Load Type", ""], ["Empty Dryer Cold Weight", ""], ["Serial Number", ""], ["Build", ""], ["Heat Setting", ""], ["Dryness Setting", ""], ["Frequency", ""], ["Washer Water Temperature ( 60 ± 5°F )", ""]], new element=w312, index (col)=1 ("disabled index (col)")) -> (w285:string[][])  [unwired: 1 in]
            n141 = Build Array (concatenate)(w285, "Flow Computer Info Baro,BTUF,u,Z") -> (→"Header Data Array":string[][])
            n142 = call <vilib>:"Add State(s) to Queue__jki_lib_state_machine.vi"("State(s) in (\"\")"=w315) -> ("States Out"=w314:string)  [unwired: 14 in]
            n143 = call "Worksheet DOE Audit.vi"() -> ("DOE Data Out"=w269:T8)  [unwired: 8 in, 2 out]
            n144 = Bundle By Name(cluster=w269, "Technician"="Technician:", "Date"=w274, "Model"="Model:", "Serial"="Serial Number:", "Load Cycles"="Load Run Number:", "Exhaust"="Exhaust:", "Supply Voltage"=w266, "Washer Water Temperature ( 60 ± 5°F )"="Washer Water \nTemperature ( 60 ± 5°F ):") -> (w277:T8)
            n145 = call "Calibration.vi"("Show Front Panel"=FALSE, "error in (no error)"=w264) -> ("error out"=w263:errorcluster, "OutputData"=w262:string[][])  [unwired: 8 in]
            n146 = call "Worksheet DOE Audit.vi"("Add?"=TRUE, "Calibration Data"=w262, "DOE Data"=w277) -> ()  [unwired: 5 in, 3 out]
          }
          frame "Initialize Data File" {
            # "Your code here.\n(You can make a copy of, or modify, this frame)"
            n147 = local read "Data File Directory"() -> (w317:path)
            n148 = local read "Header Data Array"() -> (w316:string[][])
            n149 = local read "FileName"() -> (w318:path)
            n150 = call <vilib>:"Check if File or Folder Exists.vi"("path"=w317) -> ("error out"=w322:errorcluster, "file or folder exists?"=w320:bool, "dup path"=w321:path)  [unwired: 1 in, 7 out]
            n151 = case shown="False" w320 {
              tunnel: w321 -> [w332 _]
              tunnel: w322 -> [w334 w335]
              tunnel: [w333 w335] -> w319
              frame False {
                n152 = Create Folder(path (use dialog)=w332, error in=w334) -> (error out=w333:errorcluster)  [unwired: 3 out]
              }
              frame True {
              }
            }
            n153 = case shown="No Error" w319 {
              selector: w319 -> [w329 w331]
              tunnel: w316 -> [w327 _]
              tunnel: [w329 w331] -> _
              tunnel: w318 -> [w328 _]
              frame No Error {
                n154 = call-poly <vilib>:"Write To Spreadsheet File.vi"("delimiter (\\t)"="," ("delimiter (\\t)"), "2D data"=w327, "file path (dialog if empty)"=w328) -> ()  [unwired: 5 in, 1 out]
              }
              frame Error {
              }
            }
            n155 = call <vilib>:"Add State(s) to Queue__jki_lib_state_machine.vi"("State(s) in (\"\")"=w326) -> ("States Out"=w325:string)  [unwired: 14 in]
          }
          frame "Check Contents" {
            n156 = local read "Drying Cycle:"() -> (w337:string)
            n157 = local read "Exhaust:"() -> (w350:string)
            n158 = local read "Supply Voltage:"() -> (w349:string)
            n159 = Equal?(x=w337, y="Timed Dry" ("Drying Cycle:")) -> (x = y?=w336:bool)
            n160 = String Length(string=w350) -> (length=w348:i32)
            n161 = case shown="True" w336 {
              frame False {
              }
              frame True {
                n162 = local write "Dryness Setting:"("NA" ("Dryness Setting:")) -> ()
              }
            }
            n163 = String Length(string=w337) -> (length=w347:i32)
            n164 = String Length(string=w349) -> (length=w346:i32)
            n165 = Greater Than 0?(x=w348) -> (x > 0?=w343:bool)
            n166 = Greater Than 0?(x=w347) -> (x > 0?=w344:bool)
            n167 = Unbundle By Name(w340) -> ("Local?"=w339:bool)
            n168 = Greater Than 0?(x=w346) -> (x > 0?=w345:bool)
            n169 = Compound Arithmetic op=AND(w343, w344, w345) -> (w342:bool)
            n170 = case shown="True" w342 {
              tunnel: ["" w358] -> w341
              tunnel: w339 -> [_ w357]
              frame False {
                n171 = One Button Dialog(message="All Test Data Must be Filled In") -> ()  [unwired: 1 in, 1 out]
              }
              frame True {
                n172 = case shown="False" w357 {
                  tunnel: ["UI: Front Panel State >> Close\nGet Load Definition\nGet Weights\nGenerate Filename\nGenerate Header Data\nInitialize Data File\nWrite Globals\nMacro: Exit" "Get Load Definition\nGet Weights\nGenerate Filename\nGenerate Header Data\nInitialize Data File\nWrite Globals\nMacro: Exit"] -> w358
                  frame False {
                  }
                  frame True {
                  }
                }
              }
            }
            n173 = call <vilib>:"Add State(s) to Queue__jki_lib_state_machine.vi"("State(s) in Front (\"\")"=w341, "State(s) in (\"\")"=w353) -> ("States Out"=w352:string)  [unwired: 13 in]
          }
          frame "Get Weights" {
            n174 = local read "Nominal Load  Weight"() -> (w363:string)
            n175 = Fract/Exp String To Number(string=w363) -> (number=w362:dbl)  [unwired: 3 in, 1 out]
            n176 = call "Panel RMC Calculator.vi"("Scale Com Port"="Scale Com Port", "Bone Dry Wt(lbs)"=w362) -> ("Weights Out"=w364:T1)  [unwired: 13 in]
            "Weights Out" <- w364
            n177 = Bundle By Name(cluster=w366, "Weights"=w364) -> (w365:T4)
            n178 = call <vilib>:"Add State(s) to Queue__jki_lib_state_machine.vi"("State(s) in (\"\")"=w369) -> ("States Out"=w368:string)  [unwired: 14 in]
          }
          frame "Get Load Definition" {
            n179 = call "Panel Get Load Info.vi"("file path (dialog if empty)"="Load Definition File") -> ("Load Type Out"=→"Load Type":string, "Nominal Load  Weight Out"=→"Nominal Load  Weight":string)  [unwired: 13 in]
            n180 = call <vilib>:"Add State(s) to Queue__jki_lib_state_machine.vi"("State(s) in (\"\")"=w376) -> ("States Out"=w375:string)  [unwired: 14 in]
          }
        }
      }
    }
    frame Error {
    }
  }
  n181 = Unbundle By Name(w4) -> ("Error Flag"=w3:bool)
  n182 = case shown="False" w3 {
    tunnel: [w378 w379] -> w2
    tunnel: w1 -> [w378 _]
    frame False {
    }
    frame True {
      n183 = local read "Unhandled Error"() -> (w379:errorcluster)
    }
  }
  "error out" <- w2
